vi "DPO_7K_Get_Channel_Scale.vi"(8 "Error In":errorcluster, 10 "Channel":u16(ring) items=["Channel 1", "Channel 2", "Channel 3", "Channel 4", "Math 1", "Math 2", "Math 3", "Math 4", "Reference 1", "Reference 2", "Reference 3", "Reference 4"], 11 "VISA resource name in":refnum<visa-resource-name>) -> (0 "Error Out":errorcluster, 2 "Channel Scale":dbl, 3 "VISA resource name out":refnum<visa-resource-name>)   [LabVIEW 2020]
uses:
  subVI/Set_Configuration.ctl
  subVI/Return_To_Interface.ctl
panel:
  in  "Return to Interface":T1
  in  "Set":T2
  # "GET CHANNEL SCALE"
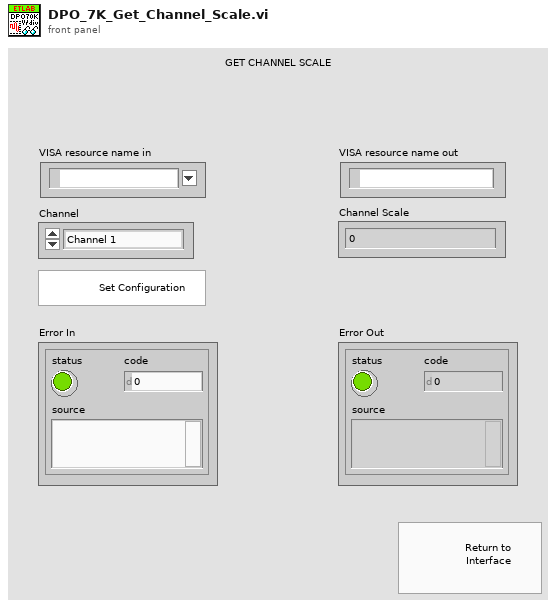
[diagram p1: front panel]
types:
  T1 = typedef "Return_To_Interface.ctl" = bool
  T2 = typedef "Set_Configuration.ctl" = bool
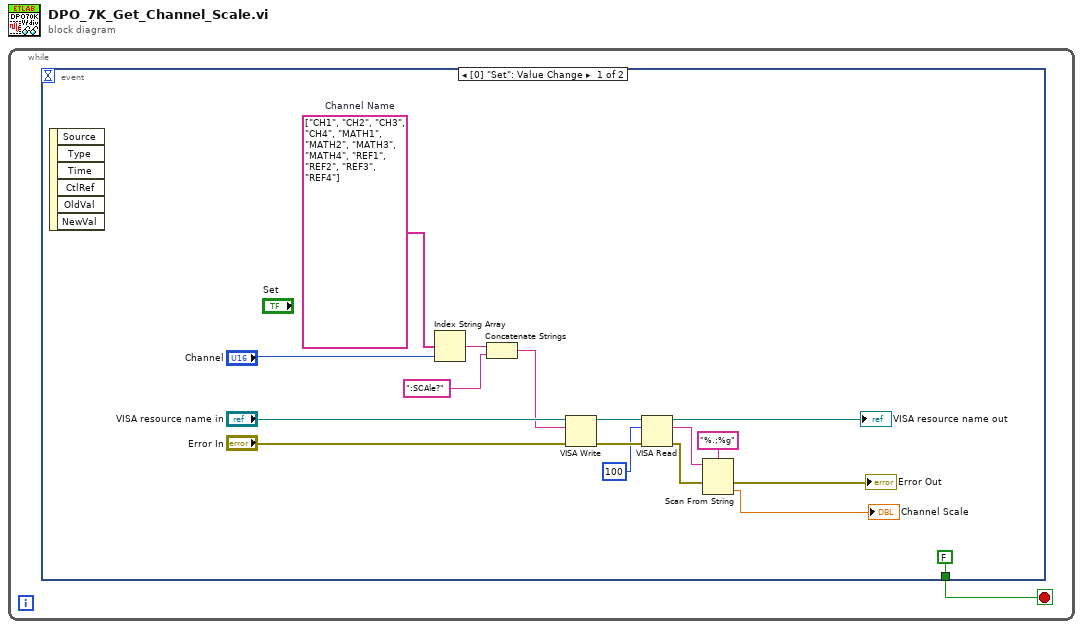
[diagram p0: block diagram]
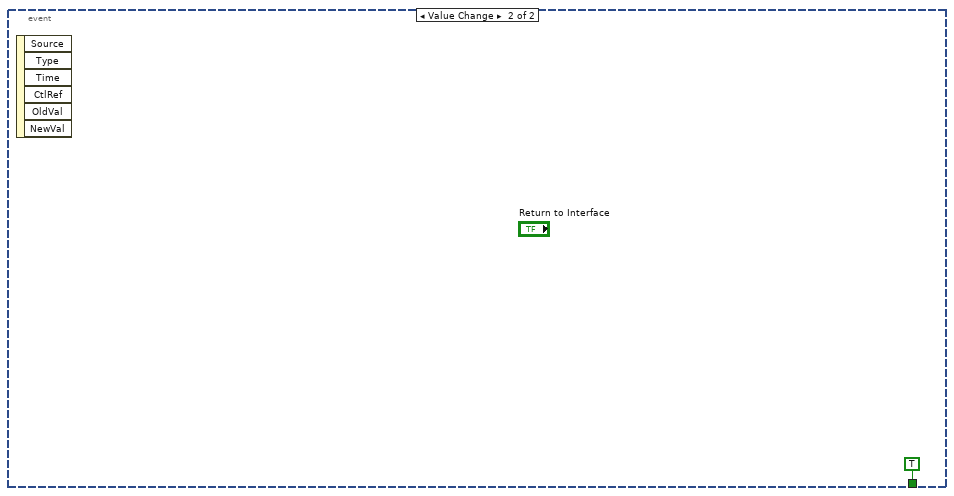
[diagram p2: hidden frame]
diagram:
  n1 = while {
    stop <- w1 stop-if-true
    n2 = event shown="[0] \"Set\": Value Change" {
      selector: _ -> [_ _]
      dyn-events: _ -> [_ _]
      timeout: _ -> [_ _]
      tunnel: [FALSE TRUE] -> w1
      event Value Change {
        w15 = string[] ["CH1", "CH2", "CH3", "CH4", "MATH1", "MATH2", "MATH3", "MATH4", "REF1", "REF2", "REF3", "REF4"]  # Channel Name
        n3 = event-data() -> ()  [unwired: 1 in, 6 out]
        n4 = Index String Array(1:"Channel", 2:w15) -> (0:w5:string)  [unwired: 1 in]
        n5 = Concatenate Strings(w5, ":SCAle?") -> (w3:string)
        n6 = VISA Write(VISA resource name="VISA resource name in", write buffer=w3, error in (no error)="Error In") -> (VISA resource name out=w13:refnum<visa-resource-name>, error out=w12:errorcluster)  [unwired: 1 out]
        n7 = VISA Read(VISA resource name=w13, byte count=u32 100, error in (no error)=w12) -> (VISA resource name out=→"VISA resource name out":refnum<visa-resource-name>, read buffer=w9:string, error out=w10:errorcluster)  [unwired: 1 out]
        n8 = Scan From String(format string="%.;%g", input string=w9, error in=w10) -> (error out=→"Error Out":errorcluster, output 1=→"Channel Scale":dbl)  [unwired: 2 in, 2 out]
      }
      event Value Change {
        n9 = event-data() -> ()  [unwired: 1 in, 6 out]
      }
    }
  }
